vi "Gear Control.vi"(6 "Boolean":bool, 9 "Gear speed":dbl=2.0, 10 "Axes 2":dbl[](array[numeric]), 11 "Axes":dbl[](array[numeric])) -> (1 "Output":bool, 2 "upper limit":dbl, 3 "Control Mode":T1)   [LabVIEW 2016]
uses:
  <vilib>/Rock Robotics/WPI/ThirdParty/CanMotor/TalonSRX/WPI_CANTalonSRX_APIControlMode.ctl
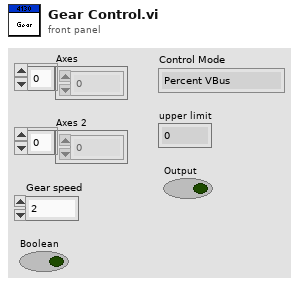
[diagram p1: front panel]
types:
  T1 = typedef "WPI_CANTalonSRX_APIControlMode.ctl" = enum8{"Percent VBus", "Speed", "Position", "Slave", "Unchanged / Invalid", "Voltage Compensation", "Current", "Motion Profile", "Motion Magic"}
  T2 = typedef "WPI_DigitalInputDevRef.ctl" = cluster{"DevStatus":errorcluster, "DIO Channel":T3}
  T3 = typedef "FPGA_DIOChannel.ctl" = enum8{"DIO 0", "DIO 1", "DIO 2", "DIO 3", "DIO 4", "DIO 5", "DIO 6", "DIO 7", "DIO 8", "DIO 9", "DIO MXP 0", "DIO MXP 1", "DIO MXP 2", "DIO MXP 3", "DIO MXP 4", "DIO MXP 5", "DIO MXP 6", "DIO MXP 7", "DIO MXP 8", "DIO MXP 9", "DIO MXP 10", "DIO MXP 11", "DIO MXP 12", "DIO MXP 13", "DIO MXP 14", "DIO MXP 15", "SPI Port CS1", "SPI Port CS2", "SPI Port CS3", "SPI Port MISO", "SPI Port MOSI", "Invalid"}
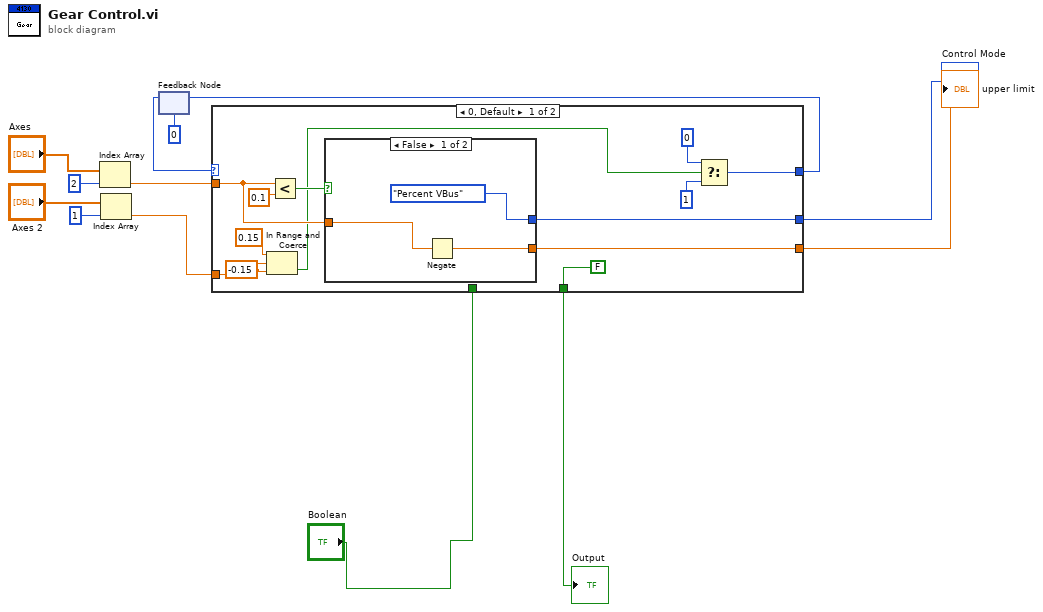
[diagram p0: block diagram]
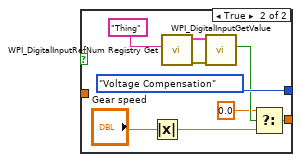
[diagram p2: hidden frame]
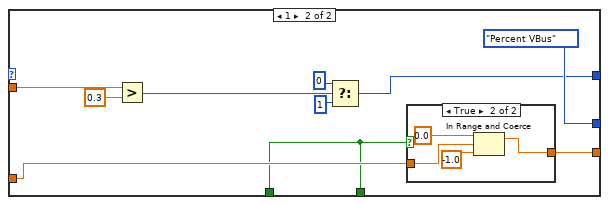
[diagram p3: hidden frame]
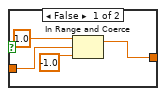
[diagram p4: hidden frame]
diagram:
  n1 = Index Array(array="Axes", index=2) -> (element=w8:dbl)
  n2 = Index Array(array="Axes 2", index=1) -> (element=w10:dbl)
  n3 = feedback #1(0) -> (w5:i32)
  n4 = case shown="0, Default" w5 {
    tunnel: [w22 w43] -> w4
    tunnel: [w26 WPI_CANTalonSRX_APIControlMode."Percent VBus" ("Control Mode")] -> w7
    tunnel: w8 -> [w23 w46]
    tunnel: [w15 w40] -> w9
    tunnel: w10 -> [w19 w47]
    tunnel: "Boolean" -> [_ w39]
    tunnel: [FALSE ("Output") w39] -> w13
    frame 0, Default {
      n5 = In Range and Coerce(upper limit=0.15, x=w19, lower limit=-0.15) -> (In Range?=w16:bool)  [unwired: 1 out]
      n6 = Less?(x=w23, y=0.1) -> (x < y?=w24:bool)
      n7 = case shown="False" w24 {
        tunnel: [WPI_CANTalonSRX_APIControlMode."Percent VBus" ("Control Mode") WPI_CANTalonSRX_APIControlMode."Voltage Compensation" ("Control Mode")] -> w26
        tunnel: [w27 w31] -> w15
        tunnel: w23 -> [w28 _]
        frame False {
          n8 = Negate(x=w28) -> (-x=w27:dbl)
        }
        frame True {
          n9 = Absolute Value(x="Gear speed") -> (abs(x)=w30:dbl)
          n10 = call <vilib>:"WPI_DigitalInputRefNum Registry Get.vi"("refnum name"="Thing") -> ("error out"=w36:errorcluster, "DigitalInputDevRef"=w37:T2)  [unwired: 9 in]
          n11 = call <vilib>:"WPI_DigitalInputGetValue.vi"("error in (no error)"=w36, "DigitalInputDevRef"=w37) -> ("Value"=w34:bool)  [unwired: 7 in, 2 out]
          n12 = Select(t=0.0, s=w34, f=w30) -> (s? t:f=w31:dbl)
        }
      }
      n13 = Select(t=0, s=w16, f=1) -> (s? t:f=w22:i32)
    }
    frame 1 {
      n14 = Greater?(x=w46, y=0.3) -> (0:w44:bool)
      n15 = Select(t=0, s=w44, f=1) -> (s? t:f=w43:i32)
      n16 = case shown="True" w39 {
        tunnel: [w52 w56] -> w40
        tunnel: w47 -> [w51 w55]
        frame False {
          n17 = In Range and Coerce(upper limit=1.0, x=w51, lower limit=-1.0) -> (coerced(x)=w52:dbl)  [unwired: 1 out]
        }
        frame True {
          n18 = In Range and Coerce(upper limit=0.0, x=w55, lower limit=-1.0) -> (coerced(x)=w56:dbl)  [unwired: 1 out]
        }
      }
    }
  }
  "Output" <- w13
  "upper limit" <- w9
  "Control Mode" <- w7
  n19 = feedback-in #1(w4) -> ()
